vi "PV ActiveLine - Example Read Data.vi"(7 "Baud Rate":u32(ring) items=["9600 (default)", "19200", "38400", "57600", "115200"], 8 "error in (no error)":errorcluster caption="Fehler (Eingang, kein Fehler)", 11 "input refnum":refnum<visa-resource-name> caption="Eingang (Referenz)") -> (0 "error out":errorcluster, 1 "Programversion":string, 2 "Device Type":string)   [LabVIEW 2013, in "PV ActiveLine.lvlib"]
doc: "This VI is an example of how to use the PV ActiveLine subVIs programmatically. This VI first initializes the instrument, takes measurements, then closes the instrument."
uses:
  C:/Program Files (x86)/National Instruments/LabVIEW 2013/PV ActiveLine/PV ActiveLine.lvlib
  Public/Configure/PV ActiveLine - FullScaleRange (TPG361).vi
  Public/Configure/PV ActiveLine - FullScaleRange (TPG362).vi
  Public/Configure/PV ActiveLine - FilterTime (TPG361).vi
  Public/Configure/PV ActiveLine - FilterTime (TPG362).vi
  Public/Configure/PV ActiveLine - CalibrationFactor (TPG361).vi
  Public/Configure/PV ActiveLine - CalibrationFactor (TPG362).vi
panel:
  out "Get Calibration factor 1":dbl=0.000753 format="%.3f"
  out "Get Calibration factor 2":dbl=0.000753 format="%.3f"
  out "Sensor 2 Get":i8(ring)=3 items=["0.01 mbar", "0.1 mbar", "1 mbar", "10 mbar", "100 mbar", "1000 mbar", "2 bar", "5 bar", "10 bar", "50 bar"]
  out "Sensor 1 Get":i8(ring)=3 items=["0.01 mbar", "0.1 mbar", "1 mbar", "10 mbar", "100 mbar", "1000 mbar", "2 bar", "5 bar", "10 bar", "50 bar"]
  out "Sensor 1 Get 2":i8(ring)=2 items=["Filter off", "fast", "normal", "slow"]
  out "Sensor 2 Get 2":i8(ring)=2 items=["Filter off", "fast", "normal", "slow"]
  out "Unit Get":i8(ring) items=["mbar / bar", "Torr", "Pascal", "Micron", "hPascal (default)", "Volt"]
  in  "Unit Set":i8(ring) items=["mbar / bar", "Torr", "Pascal", "Micron", "hPascal (default)", "Volt"]
  out "Sensor 2":string
  out "Sensor 1":string
  in  "W/R":bool
  out "Status Sensor 2":i32(ring) items=["data OK", "underrange", "overrange", "sensor error", "sensor off", "no sensor", "ID error"]
  out "Status Sensor 1":i32(ring) items=["data OK", "underrange", "overrange", "sensor error", "sensor off", "no sensor", "ID error"]
  out "Pressure Sensor 2":dbl format="%.3e"
  out "Pressure Sensor 1":dbl format="%.3e"
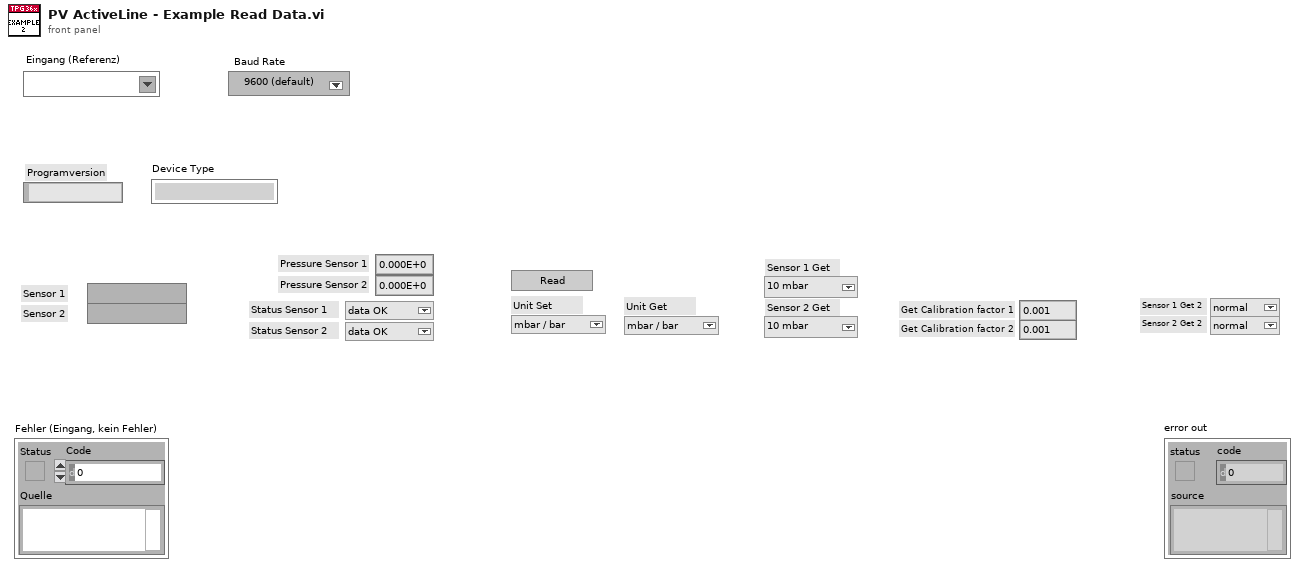
[diagram p1: front panel]
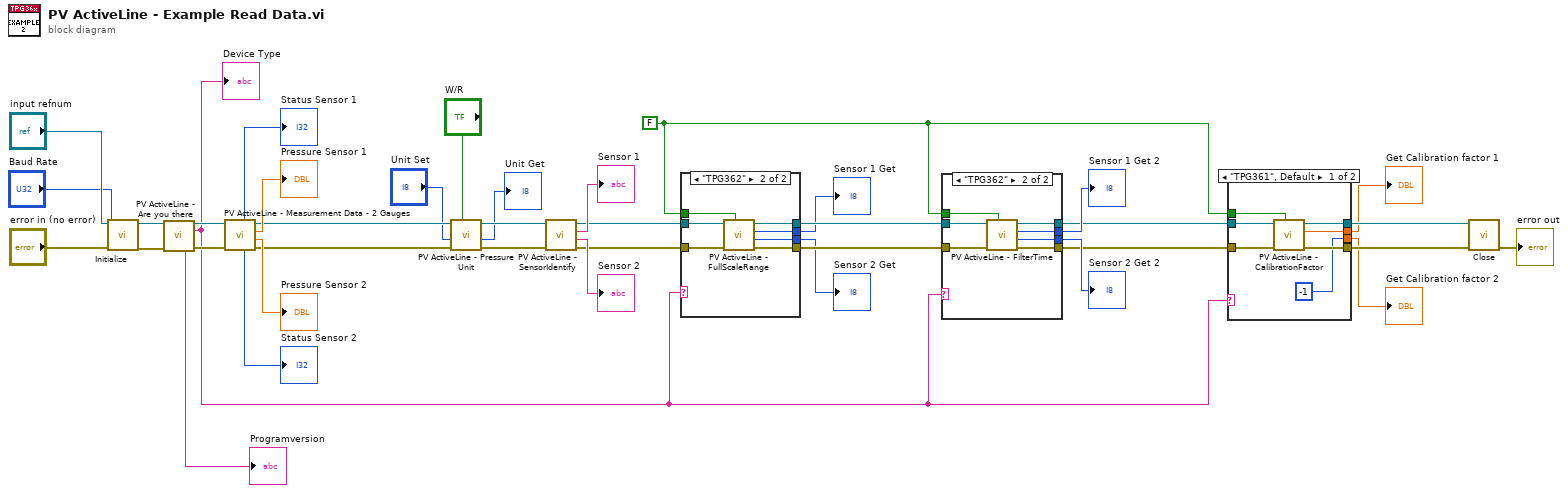
[diagram p0: block diagram]
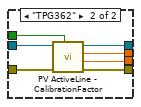
[diagram p2: hidden frame]
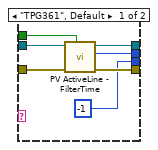
[diagram p3: hidden frame]
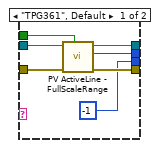
[diagram p4: hidden frame]
diagram:
  w11 = FALSE ("W/R")
  n1 = call "Initialize.vi"("error in (no error)"="error in (no error)", "Baud Rate"="Baud Rate", "input refnum"="input refnum") -> ("Cluster (Ausgang)"=w5:errorcluster, "Referenz out"=w8:refnum<visa-resource-name>)  [unwired: 7 in]
  n2 = call "PV ActiveLine - Are you there.vi"("Referenz in"=w8, "Fehler (Eingang)"=w5) -> ("Referenz out"=w7:refnum<visa-resource-name>, "Device Type"=w3:string, "Firmware Version"=→"Programversion":string, "Cluster (Ausgang)"=w6:errorcluster)  [unwired: 7 in, 3 out]
  "Device Type" <- w3
  n3 = call "PV ActiveLine - Measurement Data - 2 Gauges.vi"("Fehler (Eingang)"=w6, "Referenz in"=w7) -> ("Cluster (Ausgang)"=w30:errorcluster, "Pressure Sensor 2"=→"Pressure Sensor 2":dbl, "Pressure Sensor 1"=→"Pressure Sensor 1":dbl, "Referenz out"=w31:refnum<visa-resource-name>, "Status Sensor 2"=→"Status Sensor 2":i32, "Status Sensor 1"=→"Status Sensor 1":i32)  [unwired: 4 in]
  n4 = call "PV ActiveLine - Pressure Unit.vi"("W/R"="W/R", "Fehler (Eingang)"=w30, "Unit Set"="Unit Set", "Referenz in"=w31) -> ("Cluster (Ausgang)"=w27:errorcluster, "Unit Get"=→"Unit Get":i8, "Referenz out"=w28:refnum<visa-resource-name>)  [unwired: 5 in]
  n5 = call "PV ActiveLine - SensorIdentify.vi"("Fehler (Eingang)"=w27, "Referenz in"=w28) -> ("Cluster (Ausgang)"=w13:errorcluster, "Sensor 2"=→"Sensor 2":string, "Sensor 1"=→"Sensor 1":string, "Referenz out"=w15:refnum<visa-resource-name>)  [unwired: 6 in]
  n6 = case shown="\"TPG362\"" w3 {
    tunnel: w15 -> [w45 w52]
    tunnel: [w44 w51] -> w14
    tunnel: w13 -> [w43 w50]
    tunnel: [w42 w49] -> w12
    tunnel: w11 -> [w41 w48]
    tunnel: [w40 w47] -> w10
    tunnel: [-1 w46] -> w9
    frame "TPG361", Default {
      n7 = call-poly "PV ActiveLine - FullScaleRange.vi"("W/R"=w41, "Fehler (Eingang)"=w43, "Referenz in"=w45) -> ("Cluster (Ausgang)"=w42:errorcluster, "Sensor 1 Get"=w40:i8, "Referenz out"=w44:refnum<visa-resource-name>)  [unwired: 6 in]
    }
    frame "TPG362" {
      n8 = call-poly "PV ActiveLine - FullScaleRange.vi"("W/R"=w48, "Fehler (Eingang)"=w50, "Referenz in"=w52) -> ("Cluster (Ausgang)"=w49:errorcluster, "Sensor 2 Get"=w46:i8, "Sensor 1 Get"=w47:i8, "Referenz out"=w51:refnum<visa-resource-name>)  [unwired: 5 in]
    }
  }
  "Sensor 1 Get" <- w10
  "Sensor 2 Get" <- w9
  n9 = case shown="\"TPG362\"" w3 {
    tunnel: [-1 w61] -> w21
    tunnel: [w59 w62] -> w20
    tunnel: [w58 w65] -> w19
    tunnel: [w57 w63] -> w17
    tunnel: w14 -> [w56 w66]
    tunnel: w12 -> [w55 w64]
    tunnel: w11 -> [w54 w60]
    frame "TPG361", Default {
      n10 = call-poly "PV ActiveLine - FilterTime.vi"("W/R"=w54, "Fehler (Eingang)"=w55, "Referenz in"=w56) -> ("Cluster (Ausgang)"=w57:errorcluster, "Sensor 1 Get"=w59:i8, "Referenz out"=w58:refnum<visa-resource-name>)  [unwired: 6 in]
    }
    frame "TPG362" {
      n11 = call-poly "PV ActiveLine - FilterTime.vi"("W/R"=w60, "Fehler (Eingang)"=w64, "Referenz in"=w66) -> ("Cluster (Ausgang)"=w63:errorcluster, "Sensor 2 Get"=w61:i8, "Sensor 1 Get"=w62:i8, "Referenz out"=w65:refnum<visa-resource-name>)  [unwired: 5 in]
    }
  }
  "Sensor 2 Get 2" <- w21
  "Sensor 1 Get 2" <- w20
  n12 = case shown="\"TPG361\", Default" w3 {
    tunnel: w19 -> [w73 w80]
    tunnel: [w72 w79] -> w18
    tunnel: w17 -> [w71 w78]
    tunnel: [w70 w77] -> w16
    tunnel: w11 -> [w69 w76]
    tunnel: [w68 w75] -> w1
    tunnel: [-1 w74] -> w2
    frame "TPG361", Default {
      n13 = call-poly "PV ActiveLine - CalibrationFactor.vi"("W/R"=w69, "Fehler (Eingang)"=w71, "Referenz in"=w73) -> ("Cluster (Ausgang)"=w70:errorcluster, "Get Calibration factor 1"=w68:dbl, "Referenz out"=w72:refnum<visa-resource-name>)  [unwired: 6 in]
    }
    frame "TPG362" {
      n14 = call-poly "PV ActiveLine - CalibrationFactor.vi"("W/R"=w76, "Fehler (Eingang)"=w78, "Referenz in"=w80) -> ("Cluster (Ausgang)"=w77:errorcluster, "Get Calibration factor 2"=w74:dbl, "Get Calibration factor 1"=w75:dbl, "Referenz out"=w79:refnum<visa-resource-name>)  [unwired: 5 in]
    }
  }
  "Get Calibration factor 2" <- w2
  "Get Calibration factor 1" <- w1
  n15 = call "Close.vi"("error in (no error)"=w16, "VISA resource name"=w18) -> ("error out"=→"error out":errorcluster)  [unwired: 9 in]
